vi "Ammeter Measure (648X).vi"(8 "error in (no error)":errorcluster, 10 "Source (Function)":u16(ring) items=["Function", "Calculation 1", "Calculation 2", "Calculation 3"], 11 "VISA resource name in":refnum<visa-resource-name>) -> (0 "error out":errorcluster, 2 "Measurement":dbl, 3 "VISA resource name out":refnum<visa-resource-name>)   [LabVIEW 2016, in "Hall Effect Library.lvlib"]
uses:
  Hall Effect Library.lvlib
  <instrlib>/Keithley 648X/Keithley 648X.lvlib
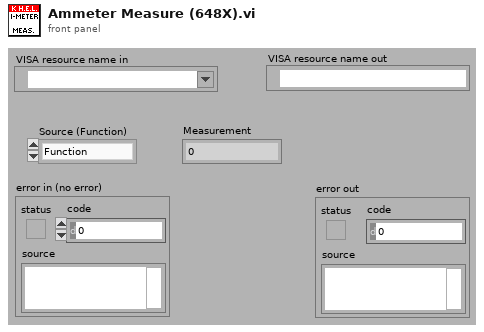
[diagram p1: front panel]
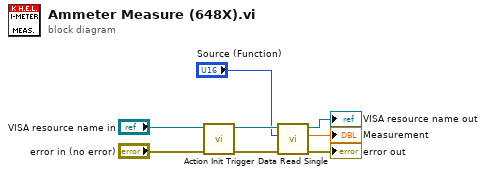
[diagram p0: block diagram]
diagram:
  n1 = call <instrlib>:"Action Init Trigger.vi"("error in (no error)"="error in (no error)", "VISA resource name"="VISA resource name in") -> ("error out"=w7:errorcluster, "VISA resource name out"=w8:refnum<visa-resource-name>)  [unwired: 8 out]
  n2 = call <instrlib>:"Data Read Single.vi"("error in"=w7, "Source (Function)"="Source (Function)", "VISA resource name"=w8) -> ("error out"=→"error out":errorcluster, "Measurement"=→"Measurement":dbl, "VISA resource name out"=→"VISA resource name out":refnum<visa-resource-name>)  [unwired: 6 out]
